vi "Adaptive Filter sim.vi"() -> ()   [LabVIEW 2017]
panel:
  in  "Rescale":bool
  in  "Decimate":bool
  out "Gradients":dbl[][](graph)
  in  "Filter":bool
  in  "Filter Size":i32=100
  out "Weights":dbl[][](graph)
  out "Taps":dbl[][](graph)
  in  "Beta":fxp<+/-,32,-16>=7.629394527697286e-06
  out "ECG Data":dbl[][](graph)
  in  "File Path Control":path=path "C:/Users/pursley/Documents/Projects/NHLBI/Lederman/Testing/2014-03-21/FL1.txt"
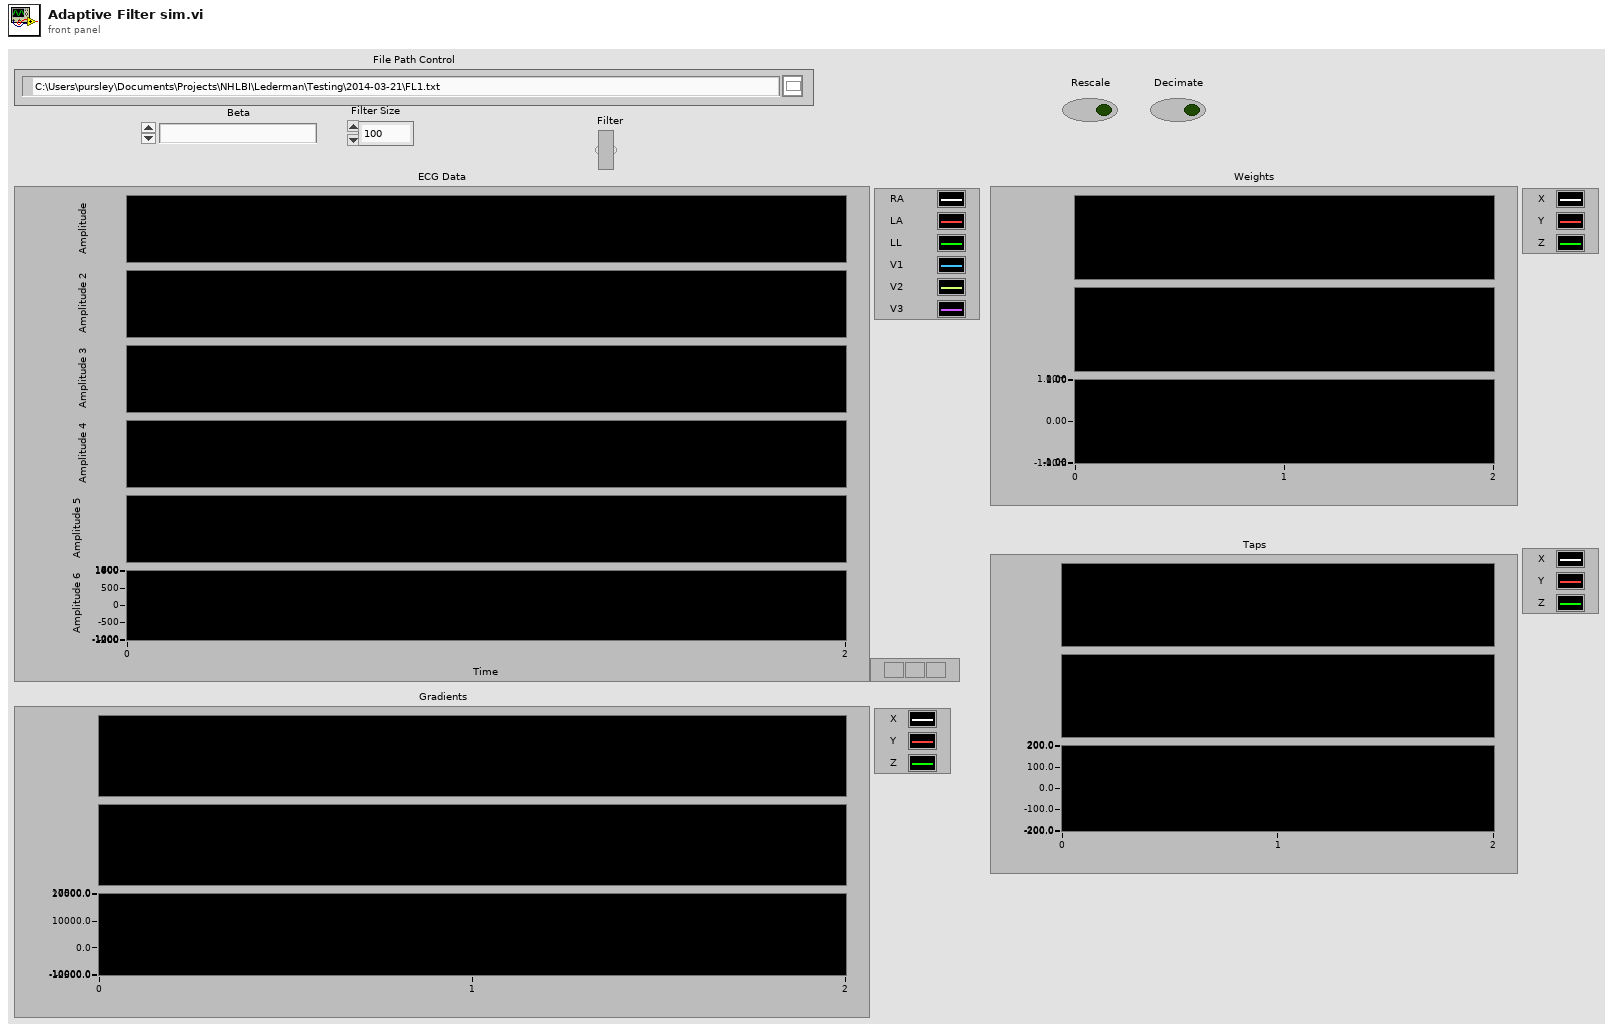
[diagram p1: front panel]
types:
  T1 = cluster{"fixed-point type":fxp<+/-,16,16>, "fixed-point type":fxp<+/-,16,16>, "fixed-point type":fxp<+/-,16,16>}
  T2 = cluster{"fixed-point type":dbl, "fixed-point type":dbl, "fixed-point type":dbl}
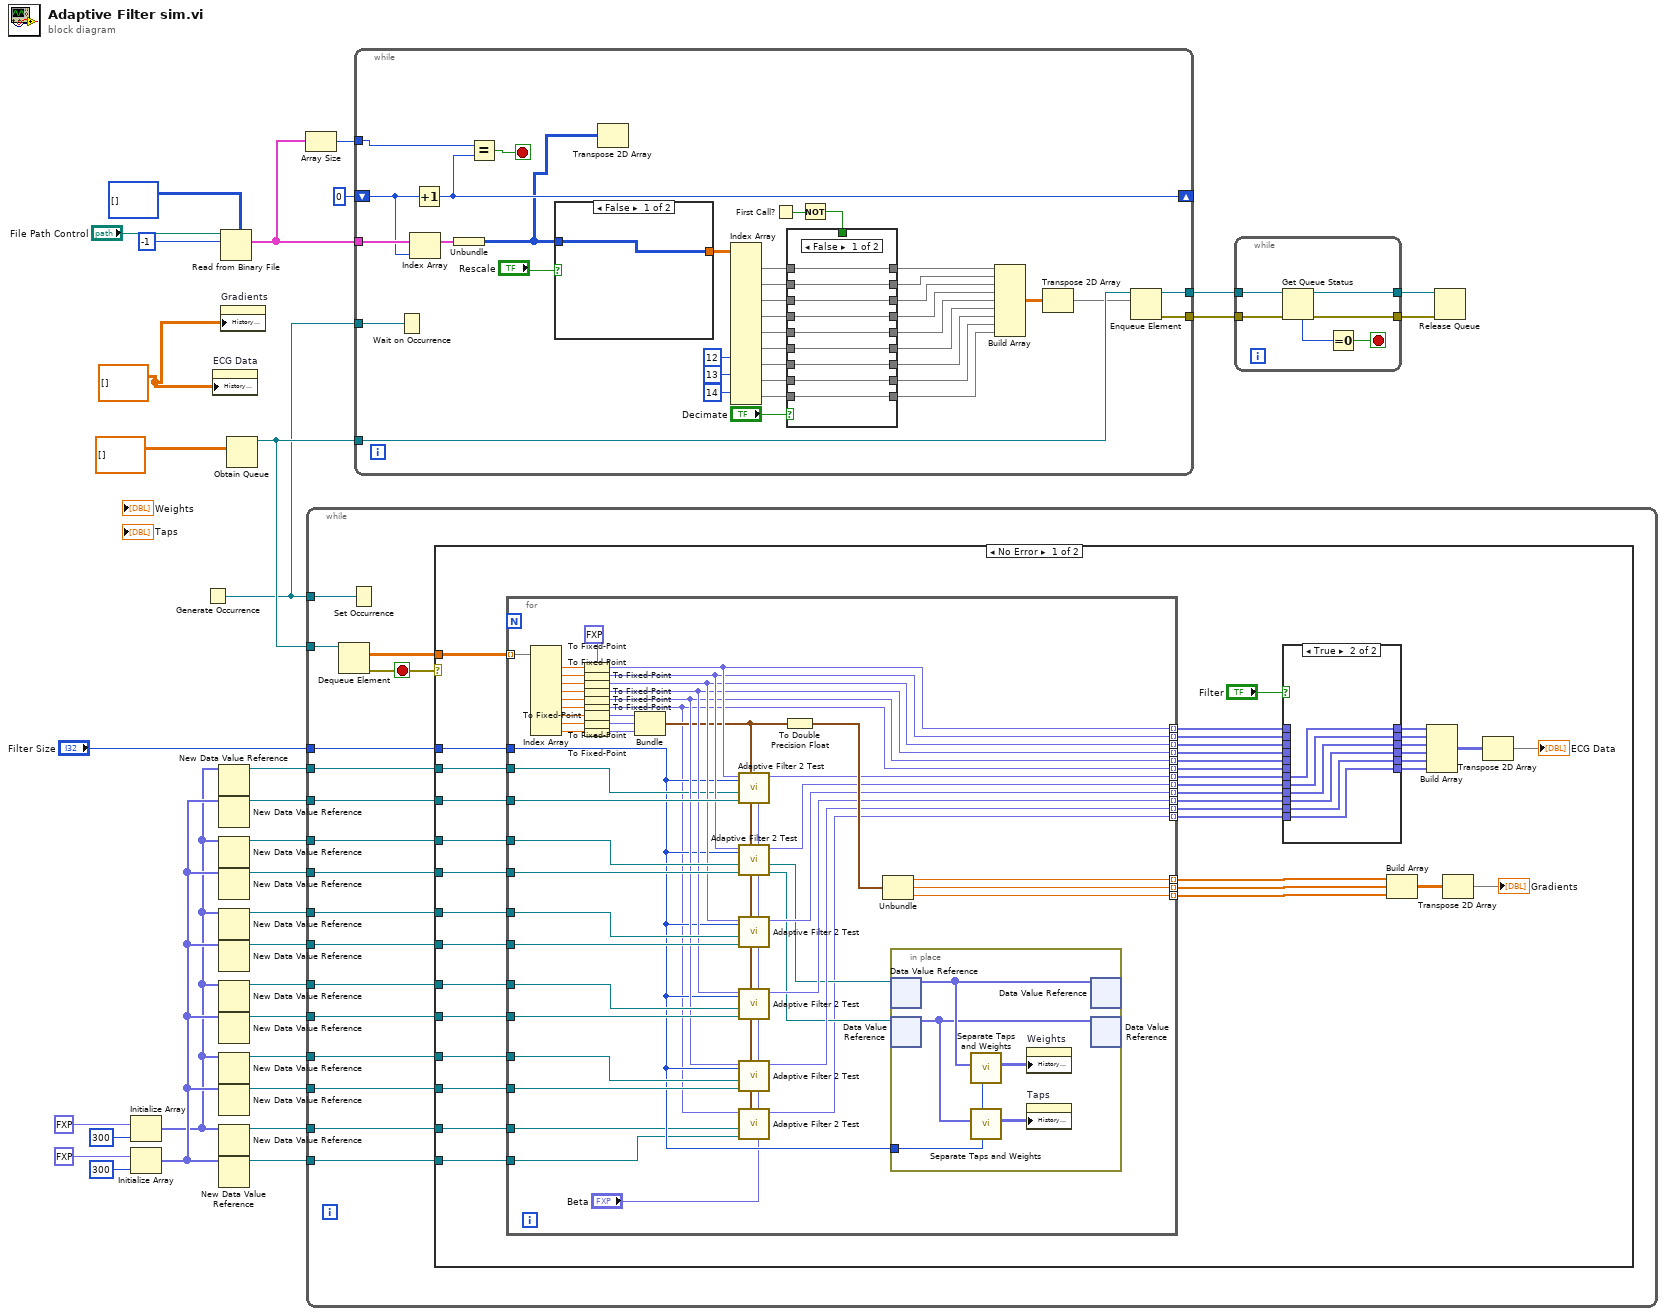
[diagram p0: block diagram]
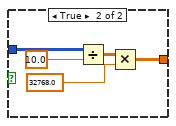
[diagram p4: hidden frame]
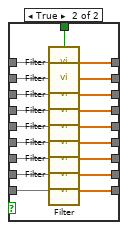
[diagram p5: hidden frame]
diagram:
  w6 = dbl[][] [] ("History Data")
  n1 = Initialize Array(fxp<+/-,24,8> 0.0 ("Z"), 300 ("dimension size")) -> (w13:fxp<+/-,24,8>[])
  n2 = Initialize Array(fxp<+/-,16,16> 0.0 ("Z"), 300 ("dimension size")) -> (w16:fxp<+/-,16,16>[])
  n3 = Generate Occurrence() -> (w7:refnum<k4>)
  n4 = property on="ECG Data" class="WFChart (strict)"("History Data"=w6) -> ()  [unwired: 2 in, 2 out]
  n5 = New Data Value Reference(data value=w13) -> (data value reference=w30:refnum<data-value>)  [unwired: 1 in, 1 out]
  n6 = New Data Value Reference(data value=w16) -> (data value reference=w29:refnum<data-value>)  [unwired: 1 in, 1 out]
  n7 = New Data Value Reference(data value=w13) -> (data value reference=w27:refnum<data-value>)  [unwired: 1 in, 1 out]
  n8 = New Data Value Reference(data value=w16) -> (data value reference=w28:refnum<data-value>)  [unwired: 1 in, 1 out]
  n9 = New Data Value Reference(data value=w13) -> (data value reference=w25:refnum<data-value>)  [unwired: 1 in, 1 out]
  n10 = New Data Value Reference(data value=w16) -> (data value reference=w26:refnum<data-value>)  [unwired: 1 in, 1 out]
  n11 = New Data Value Reference(data value=w13) -> (data value reference=w23:refnum<data-value>)  [unwired: 1 in, 1 out]
  n12 = New Data Value Reference(data value=w16) -> (data value reference=w24:refnum<data-value>)  [unwired: 1 in, 1 out]
  n13 = New Data Value Reference(data value=w13) -> (data value reference=w21:refnum<data-value>)  [unwired: 1 in, 1 out]
  n14 = New Data Value Reference(data value=w16) -> (data value reference=w22:refnum<data-value>)  [unwired: 1 in, 1 out]
  n15 = New Data Value Reference(data value=w13) -> (data value reference=w19:refnum<data-value>)  [unwired: 1 in, 1 out]
  n16 = New Data Value Reference(data value=w16) -> (data value reference=w20:refnum<data-value>)  [unwired: 1 in, 1 out]
  n17 = Read from Binary File(5:i16[][] [], 10:-1 ("count (1)"), 11:"File Path Control") -> (2:w2:cluster{i16[][]}[])  [unwired: 3 in, 3 out]
  n18 = property on="Gradients" class="WFChart (strict)"("History Data"=w6) -> ()  [unwired: 2 in, 2 out]
  n19 = Obtain Queue(element data type=dbl[][] [] ("History Data")) -> (queue out=w31:refnum<queue>)  [unwired: 4 in, 2 out]
  n20 = Array Size(array=w2) -> (size(s)=w1:i32)
  n21 = while {
    tunnel: w31 -> [w34]
    tunnel: w30 -> [w48]
    tunnel: w29 -> [w47]
    tunnel: w28 -> [w46]
    tunnel: w27 -> [w45]
    tunnel: w26 -> [w44]
    tunnel: w25 -> [w43]
    tunnel: w24 -> [w42]
    tunnel: w23 -> [w41]
    tunnel: w22 -> [w40]
    tunnel: w21 -> [w39]
    tunnel: w20 -> [w38]
    tunnel: w19 -> [w37]
    tunnel: "Filter Size" -> [w36]
    tunnel: w7 -> [w35]
    stop <- w50 stop-if-true
    n22 = Dequeue Element(queue=w34) -> (element=w49:dbl[][], error out=w50:errorcluster)  [unwired: 2 in, 2 out]
    n23 = Set Occurrence(w35) -> ()
    n24 = case shown="No Error" w50 {
      tunnel: w49 -> [w90 _]
      tunnel: w48 -> [w89 _]
      tunnel: w47 -> [w88 _]
      tunnel: w46 -> [w87 _]
      tunnel: w45 -> [w86 _]
      tunnel: w44 -> [w85 _]
      tunnel: w43 -> [w84 _]
      tunnel: w42 -> [w83 _]
      tunnel: w41 -> [w82 _]
      tunnel: w40 -> [w81 _]
      tunnel: w39 -> [w80 _]
      tunnel: w38 -> [w79 _]
      tunnel: w37 -> [w78 _]
      tunnel: w36 -> [w75 _]
      frame No Error {
        n25 = for {
          tunnel: w90 -> [w149] mode=indexing
          tunnel: w89 -> [w117]
          tunnel: w88 -> [w140]
          tunnel: w87 -> [w139]
          tunnel: w86 -> [w138]
          tunnel: w85 -> [w137]
          tunnel: w84 -> [w136]
          tunnel: w83 -> [w135]
          tunnel: w82 -> [w134]
          tunnel: w81 -> [w133]
          tunnel: w80 -> [w132]
          tunnel: w79 -> [w106]
          tunnel: w78 -> [w105]
          tunnel: [w130] -> w74 mode=indexing
          tunnel: [w129] -> w73 mode=indexing
          tunnel: [w128] -> w72 mode=indexing
          tunnel: [w127] -> w71 mode=indexing
          tunnel: [w126] -> w70 mode=indexing
          tunnel: [w125] -> w69 mode=indexing
          tunnel: [w124] -> w68 mode=indexing
          tunnel: [w123] -> w67 mode=indexing
          tunnel: [w122] -> w66 mode=indexing
          tunnel: [w121] -> w65 mode=indexing
          tunnel: [w120] -> w57 mode=indexing
          tunnel: [w119] -> w56 mode=indexing
          tunnel: [w118] -> w55 mode=indexing
          tunnel: w75 -> [w116]
          tunnel: [w104] -> w52 mode=indexing
          tunnel: [w103] -> w51 mode=indexing
          w143 = fxp<+/-,16,16> 0.0 ("fixed-point type")
          n26 = Index Array(array=w149) -> (element #1=w148:dbl, element #2=w147:dbl, element #3=w146:dbl, element #4=w145:dbl, element #5=w144:dbl, element #6=w115:dbl, element #7=w114:dbl, element #8=w113:dbl, element #9=w110:dbl)  [unwired: 9 in]
          n27 = To Fixed-Point(fixed-point type=w143, number=w148) -> (fixed-point=w130:fxp<+/-,16,16>)
          n28 = To Fixed-Point(fixed-point type=w143, number=w147) -> (fixed-point=w129:fxp<+/-,16,16>)
          n29 = To Fixed-Point(fixed-point type=w143, number=w146) -> (fixed-point=w128:fxp<+/-,16,16>)
          n30 = To Fixed-Point(fixed-point type=w143, number=w145) -> (fixed-point=w127:fxp<+/-,16,16>)
          n31 = To Fixed-Point(fixed-point type=w143, number=w144) -> (fixed-point=w126:fxp<+/-,16,16>)
          n32 = To Fixed-Point(fixed-point type=w143, number=w115) -> (fixed-point=w103:fxp<+/-,16,16>)
          n33 = To Fixed-Point(fixed-point type=w143, number=w114) -> (fixed-point=w142:fxp<+/-,16,16>)
          n34 = To Fixed-Point(fixed-point type=w143, number=w113) -> (fixed-point=w141:fxp<+/-,16,16>)
          n35 = To Fixed-Point(number=w110) -> (fixed-point=w109:fxp<+/-,16,16>)  [unwired: 1 in]
          n36 = Bundle("fixed-point type"=w142, "fixed-point type"=w141, "fixed-point type"=w109) -> (w108:T1)  [unwired: 1 in]
          n37 = call "Adaptive Filter 2 Test.vi"("Beta"="Beta", "Noise"=w108, "Filter Size"=w116, "Taps In"=w140, "Weights In"=w117, "Input"=w130) -> ("Error Out"=w125:fxp<+/-,16,16>)  [unwired: 3 in, 2 out]
          n38 = call "Adaptive Filter 2 Test.vi"("Beta"="Beta", "Noise"=w108, "Filter Size"=w116, "Taps In"=w139, "Weights In"=w138, "Input"=w129) -> ("Taps Out"=w112:refnum<data-value>, "Weights Out"=w111:refnum<data-value>, "Error Out"=w124:fxp<+/-,16,16>)  [unwired: 3 in]
          n39 = call "Adaptive Filter 2 Test.vi"("Beta"="Beta", "Noise"=w108, "Filter Size"=w116, "Taps In"=w137, "Weights In"=w136, "Input"=w128) -> ("Error Out"=w123:fxp<+/-,16,16>)  [unwired: 3 in, 2 out]
          n40 = call "Adaptive Filter 2 Test.vi"("Beta"="Beta", "Noise"=w108, "Filter Size"=w116, "Taps In"=w135, "Weights In"=w134, "Input"=w127) -> ("Error Out"=w122:fxp<+/-,16,16>)  [unwired: 3 in, 2 out]
          n41 = call "Adaptive Filter 2 Test.vi"("Beta"="Beta", "Noise"=w108, "Filter Size"=w116, "Taps In"=w133, "Weights In"=w132, "Input"=w126) -> ("Error Out"=w121:fxp<+/-,16,16>)  [unwired: 3 in, 2 out]
          n42 = call "Adaptive Filter 2 Test.vi"("Beta"="Beta", "Noise"=w108, "Taps In"=w106, "Weights In"=w105, "Input"=w103) -> ("Error Out"=w104:fxp<+/-,16,16>)  [unwired: 4 in, 2 out]
          n43 = To Double Precision Float(number=w108) -> (double precision float=w131:T2)
          n44 = Unbundle(w131) -> ("fixed-point type"=w120:dbl, "fixed-point type"=w119:dbl, "fixed-point type"=w118:dbl)
          n45 = in-place {
            in-place-border: w116 -> [w152]
            n46 = in-place-dvr #1(w111) -> (w154:fxp<+/-,24,8>[])  [unwired: 1 out]
            n47 = in-place-dvr #2(w112) -> (w153:fxp<+/-,16,16>[])  [unwired: 1 out]
            n48 = call "Separate Taps and Weights.vi"("Filter Size"=w152, "Array in"=w154) -> ("Array out"=w151:fxp<+/-,24,8>[][])  [unwired: 9 in]
            n49 = call "Separate Taps and Weights.vi"("Filter Size"=w152, "Array in"=w153) -> ("Array out"=w150:fxp<+/-,24,8>[][])  [unwired: 9 in]
            n50 = property on="Weights" class="WFChart (strict)"("History Data"=w151) -> ()  [unwired: 2 in, 2 out]
            n51 = property on="Taps" class="WFChart (strict)"("History Data"=w150) -> ()  [unwired: 2 in, 2 out]
            n52 = in-place-dvr #1(w154) -> ()  [unwired: 2 out]
            n53 = in-place-dvr #2(w153) -> ()  [unwired: 2 out]
          }
        }
        n54 = case shown="True" "Filter" {
          tunnel: w74 -> [w96 _]
          tunnel: w73 -> [w95 _]
          tunnel: w72 -> [w94 _]
          tunnel: w71 -> [w93 _]
          tunnel: w70 -> [w92 _]
          tunnel: w69 -> [_ w102]
          tunnel: w68 -> [_ w101]
          tunnel: w67 -> [_ w100]
          tunnel: w66 -> [_ w99]
          tunnel: w65 -> [_ w98]
          tunnel: [w96 w102] -> w64
          tunnel: [w95 w101] -> w63
          tunnel: [w94 w100] -> w62
          tunnel: [w93 w99] -> w61
          tunnel: [w92 w98] -> w60
          tunnel: [w91 w97] -> w53
          tunnel: w52 -> [_ w97]
          tunnel: w51 -> [w91 _]
          frame False {
          }
          frame True {
          }
        }
        n55 = Build Array(w57, w56, w55) -> (w58:dbl[][])
        n56 = Build Array(w64, w63, w62, w61, w60, w53) -> (w77:fxp<+/-,16,16>[][])
        n57 = Transpose 2D Array(2D array=w58) -> (transposed array=→"Gradients":dbl[][])
        n58 = Transpose 2D Array(2D array=w77) -> (transposed array=→"ECG Data":fxp<+/-,16,16>[][])
      }
      frame Error {
      }
    }
  }
  n59 = while {
    shift-right: [w161] -> _
    shift-left: 0 ("mark after read (chars.)") -> [w163]
    tunnel: w31 -> [w173]
    tunnel: [w172] -> w12
    tunnel: [w169] -> w10
    tunnel: w7 -> [w168]
    tunnel: w2 -> [w165]
    tunnel: w1 -> [w162]
    stop <- w160 stop-if-true
    n60 = Wait on Occurrence(2:w168) -> ()  [unwired: 2 in, 1 out]
    n61 = Index Array(array=w165, index=w163) -> (element=w164:cluster{i16[][]})
    n62 = Increment(x=w163) -> (x+1=w161:i32)
    n63 = Unbundle(w164) -> (w156:i16[][])
    n64 = Equal?(x=w162, y=w161) -> (x = y?=w160:bool)
    n65 = case shown="False" "Rescale" {
      tunnel: w156 -> [w194 w199]
      tunnel: [w194 w195] -> w193
      frame False {
      }
      frame True {
        n66 = Divide(x=w199, y=10.0) -> (x/y=w197:dbl[][])
        n67 = Multiply(x=w197, y=32768.0) -> (x*y=w195:dbl[][])
      }
    }
    n68 = Transpose 2D Array(2D array=w156) -> ()  [unwired: 1 out]
    n69 = Index Array(array=w193, index (row) #7=12 ("index (row)"), index (row) #8=13 ("index (row)"), index (row) #9=14 ("index (row)")) -> (element #1=w192:dbl[], element #2=w190:dbl[], element #3=w189:dbl[], element #4=w188:dbl[], element #5=w187:dbl[], element #6=w186:dbl[], element #7=w185:dbl[], element #8=w184:dbl[], element #9=w183:dbl[])  [unwired: 15 in]
    n70 = First Call?() -> (First Call?: T/F=w191:bool)
    n71 = Not(x=w191) -> (.not. x?=w182:bool)
    n72 = case shown="False" "Decimate" {
      tunnel: w192 -> [w208 w227]
      tunnel: w190 -> [w207 w226]
      tunnel: w189 -> [w206 w225]
      tunnel: w188 -> [w205 w224]
      tunnel: w187 -> [w204 w223]
      tunnel: w186 -> [w203 w222]
      tunnel: w185 -> [w202 w221]
      tunnel: w184 -> [w201 w220]
      tunnel: w183 -> [w200 w219]
      tunnel: w182 -> [_ w218]
      tunnel: [w208 w217] -> w181
      tunnel: [w207 w216] -> w180
      tunnel: [w206 w215] -> w179
      tunnel: [w205 w214] -> w178
      tunnel: [w204 w213] -> w177
      tunnel: [w203 w212] -> w176
      tunnel: [w202 w211] -> w175
      tunnel: [w201 w210] -> w174
      tunnel: [w200 w209] -> w155
      frame False {
      }
      frame True {
        n73 = call "Filter.vi"("Array"=w227, "init/cont (init:F)"=w218) -> ("Decimated Array"=w217:dbl[])
        n74 = call "Filter.vi"("Array"=w226, "init/cont (init:F)"=w218) -> ("Decimated Array"=w216:dbl[])
        n75 = call "Filter.vi"("Array"=w225, "init/cont (init:F)"=w218) -> ("Decimated Array"=w215:dbl[])
        n76 = call "Filter.vi"("Array"=w224, "init/cont (init:F)"=w218) -> ("Decimated Array"=w214:dbl[])
        n77 = call "Filter.vi"("Array"=w223, "init/cont (init:F)"=w218) -> ("Decimated Array"=w213:dbl[])
        n78 = call "Filter.vi"("Array"=w222, "init/cont (init:F)"=w218) -> ("Decimated Array"=w212:dbl[])
        n79 = call "Filter.vi"("Array"=w221, "init/cont (init:F)"=w218) -> ("Decimated Array"=w211:dbl[])
        n80 = call "Filter.vi"("Array"=w220, "init/cont (init:F)"=w218) -> ("Decimated Array"=w210:dbl[])
        n81 = call "Filter.vi"("Array"=w219, "init/cont (init:F)"=w218) -> ("Decimated Array"=w209:dbl[])
      }
    }
    n82 = Build Array(w181, w180, w179, w178, w177, w176, w175, w174, w155) -> (w171:dbl[][])
    n83 = Transpose 2D Array(2D array=w171) -> (transposed array=w170:dbl[][])
    n84 = Enqueue Element(queue=w173, element=w170) -> (queue out=w172:refnum<queue>, error out=w169:errorcluster)  [unwired: 2 in, 1 out]
  }
  n85 = while {
    tunnel: w12 -> [w233]
    tunnel: [w232] -> w11
    tunnel: w10 -> [w231]
    tunnel: [w230] -> w9
    stop <- w228 stop-if-true
    n86 = Get Queue Status(queue=w233, error in (no error)=w231) -> (queue out=w232:refnum<queue>, error out=w230:errorcluster, # elements in queue=w229:i32)  [unwired: 1 in, 5 out]
    n87 = Equal To 0?(x=w229) -> (x = 0?=w228:bool)
  }
  n88 = Release Queue(queue=w11, error in (no error)=w9) -> ()  [unwired: 1 in, 3 out]
